vi "UNLOAD_DOOR_CLOSED_TRIGGER.vi"(7 "CYCLE DATA IN":T1, 8 "error in (no error)":errorcluster) -> (0 "error out":errorcluster, 5 "CYCLE DATA OUT":T1)   [LabVIEW 2017]
uses:
  Controls/Unload_Cyc_Data.ctl
  Controls/QUEUE_STATES.ctl
  Controls/Unload_St.ctl
  <vilib>/Utility/file.llb/Read Delimited Spreadsheet (string).vi
  <vilib>/Utility/file.llb/Write Delimited Spreadsheet (string).vi
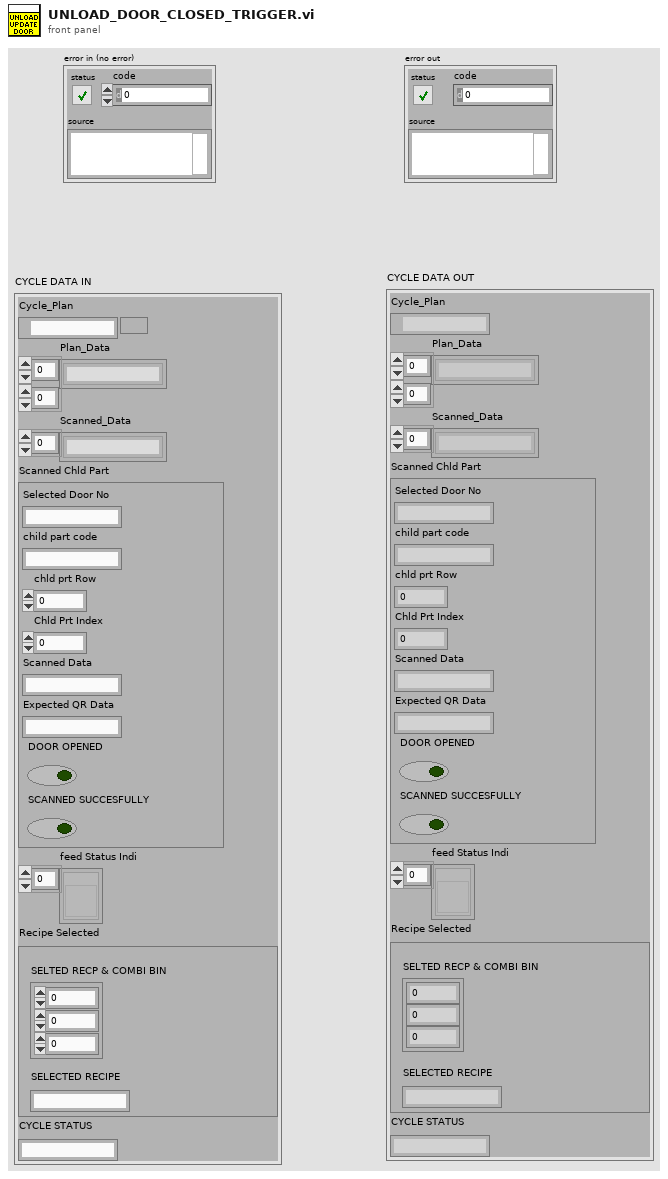
[diagram p1: front panel]
types:
  T1 = typedef "Unload_Cyc_Data.ctl" = cluster{"Cycle_Plan":path, "Plan_Data":string[][], "Scanned_Data":string[], "Scanned Chld Part":cluster{"Selected Door No":string, "child part code":string, "chld prt Row":i32, "Chld Prt Index":i32, "Scanned Data":string, "Expected QR Data":string, "DOOR OPENED":bool, "SCANNED SUCCESFULLY":bool}, "feed Status Indi":refnum<vi>[], "Recipe Selected":cluster{"SELTED RECP & COMBI BIN":cluster{"RECIPE INDEX":i32, "COMBI BIN":i32, "Section row no.":i32}, "SELECTED RECIPE":string}, "CYCLE STATUS":string}
  T2 = cluster{"RECIPE INDEX":i32, "COMBI BIN":i32, "Section row no.":i32}
  T3 = typedef "Unload_St.ctl" = enum16{"Int", "Int 2", "Wait", "Cluster_update", "Empty_Bin_Check", "Check_Section_to_Run", "Open_Door", "QR_Scanned", "Close_Door", "Error_Handler", "Stop"}
  T4 = typedef "QUEUE_STATES.ctl" = enum16{"CREATE Q", "EN Q", "DE Q", "CLOSE Q"}
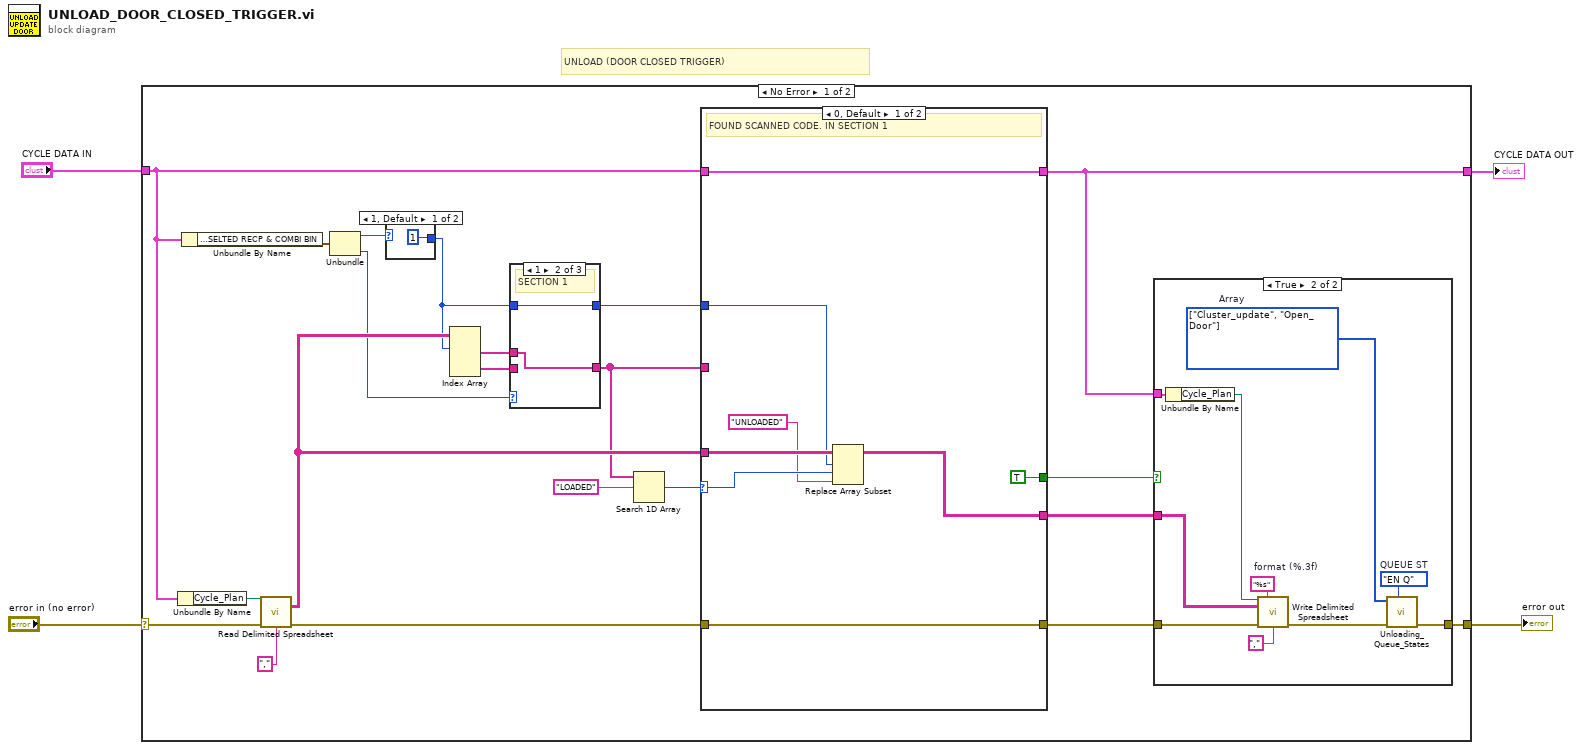
[diagram p0: block diagram]
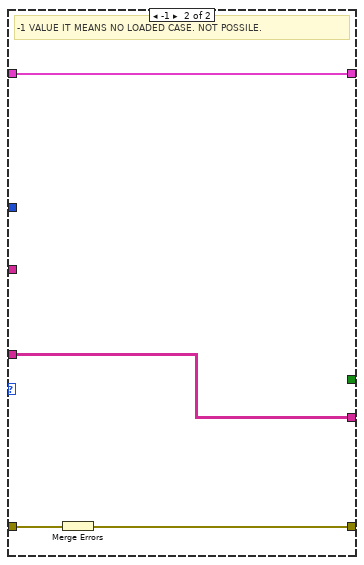
[diagram p3: hidden frame]
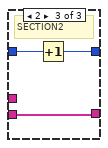
[diagram p5: hidden frame]
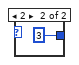
[diagram p6: hidden frame]
diagram:
  # "UNLOAD (DOOR CLOSED TRIGGER)"
  n1 = case shown="No Error" "error in (no error)" {
    selector: "error in (no error)" -> [w22 w57]
    tunnel: [w15 w57] -> w3
    tunnel: [w13 w56] -> w1
    tunnel: "CYCLE DATA IN" -> [w18 w56]
    frame No Error {
      n2 = Unbundle By Name(w18) -> ("Cycle_Plan"=w23:path)
      n3 = Unbundle By Name(w18) -> ("Recipe Selected.SELTED RECP & COMBI BIN"=w20:T2)
      n4 = call-poly <vilib>:"Read Delimited Spreadsheet.vi"("file path (dialog if empty)"=w23, "error in (no error)"=w22, "delimiter (\\t)"=",") -> ("all rows"=w16:string[][], "error out"=w21:errorcluster)  [unwired: 7 in, 4 out]
      n5 = Unbundle(w20) -> ("RECIPE INDEX"=w19:i32, "Section row no."=w10:i32)  [unwired: 1 out]
      n6 = case shown="1, Default" w19 {
        tunnel: [1 3] -> w6
        frame 1, Default {
        }
        frame 2 {
        }
      }
      n7 = Index Array(array=w16, index (row) #1=w6) -> (element #1=w9:string[], element #2=w8:string[])  [unwired: 3 in]
      n8 = case shown="1" w10 {
        tunnel: w9 -> [_ w50 _]
        tunnel: w8 -> [_ _ w53]
        tunnel: [_ w50 w53] -> w7
        tunnel: w6 -> [_ w49 w52]
        tunnel: [_ w49 w51] -> w5
        frame 0, Default {
          # "NO SECTION"
        }
        frame 1 {
          # "SECTION 1"
        }
        frame 2 {
          # "SECTION2"
          n9 = Increment(x=w52) -> (x+1=w51:i32)
        }
      }
      n10 = Search 1D Array(1D array=w7, element="LOADED") -> (index of element=w17:i32)  [unwired: 1 in]
      n11 = case shown="0, Default" w17 {
        selector: w17 -> [w39 _]
        tunnel: [w44 w45] -> w25
        tunnel: w21 -> [w44 w48]
        tunnel: [w43 w47] -> w13
        tunnel: w18 -> [w43 w47]
        tunnel: w16 -> [w40 w46]
        tunnel: w7 -> [_ _]
        tunnel: [w42 w46] -> w12
        tunnel: [TRUE _] -> w14
        tunnel: w5 -> [w37 _]
        frame 0, Default {
          # "FOUND SCANNED CODE. IN SECTION 1"
          n12 = Replace Array Subset(array=w40, new element="UNLOADED", index (row)=w37, index (col)=w39) -> (w42:string[][])
        }
        frame -1 {
          # "-1 VALUE IT MEANS NO LOADED CASE. NOT POSSILE."
          n13 = Merge Errors(w48) -> (w45:errorcluster)
        }
      }
      n14 = case shown="True" w14 {
        tunnel: w25 -> [w26 w35]
        tunnel: [w26 w27] -> w15
        tunnel: w13 -> [_ w34]
        tunnel: w12 -> [_ w31]
        frame False {
        }
        frame True {
          w29 = T3[] [enum."Cluster_update", enum."Open_Door"] items=["Int", "Int 2", "Wait", "Cluster_update", "Empty_Bin_Check", "Check_Section_to_Run", "Open_Door", "QR_Scanned", "Close_Door", "Error_Handler", "Stop"]  # Array
          w30 = QUEUE_STATES."EN Q"  # QUEUE ST
          w32 = "%s"  # format (%.3f)
          n15 = Unbundle By Name(w34) -> ("Cycle_Plan"=w33:path)
          n16 = call-poly <vilib>:"Write Delimited Spreadsheet.vi"("file path (dialog if empty)"=w33, "format (%s)"=w32, "2D data"=w31, "error in (no error)"=w35, "delimiter (\\t)"=",") -> ("error out"=w28:errorcluster)  [unwired: 9 in, 1 out]
          n17 = call "Unloading_Queue_States.vi"("QUEUE ST"=w30, "error in"=w28, "Unload St"=w29) -> ("error OUT"=w27:errorcluster)  [unwired: 7 in, 1 out]
        }
      }
    }
    frame Error {
    }
  }
  "error out" <- w3
  "CYCLE DATA OUT" <- w1
